vi "dcs_rtl_visv2.vi"() -> ()   [LabVIEW 2020]
uses:
  <vilib>/Utility/file.llb/Read Delimited Spreadsheet (DBL).vi
panel:
  out "Waveform Chart":cluster{dbl, dbl}(graph)
  out "1-D Array of Real":dbl[](array[numeric])
  out "size(s) 2":i32
  in  "milliseconds to wait":u32
  out "size(s) 4":i32[](array[numeric])
  out "Numeric":i32
  out "concatenated string":string
  out "size(s)":i32
  out "filenames":string[](array[string])
  in  "file path (dialog if empty) 2":path
  out "all rows 2":dbl[][](array[numeric])
  out "Waveform Graph 2":dbl[][](graph)
  out "Waveform Graph":dbl[][](graph)
  out "all rows":dbl[][](array[numeric])
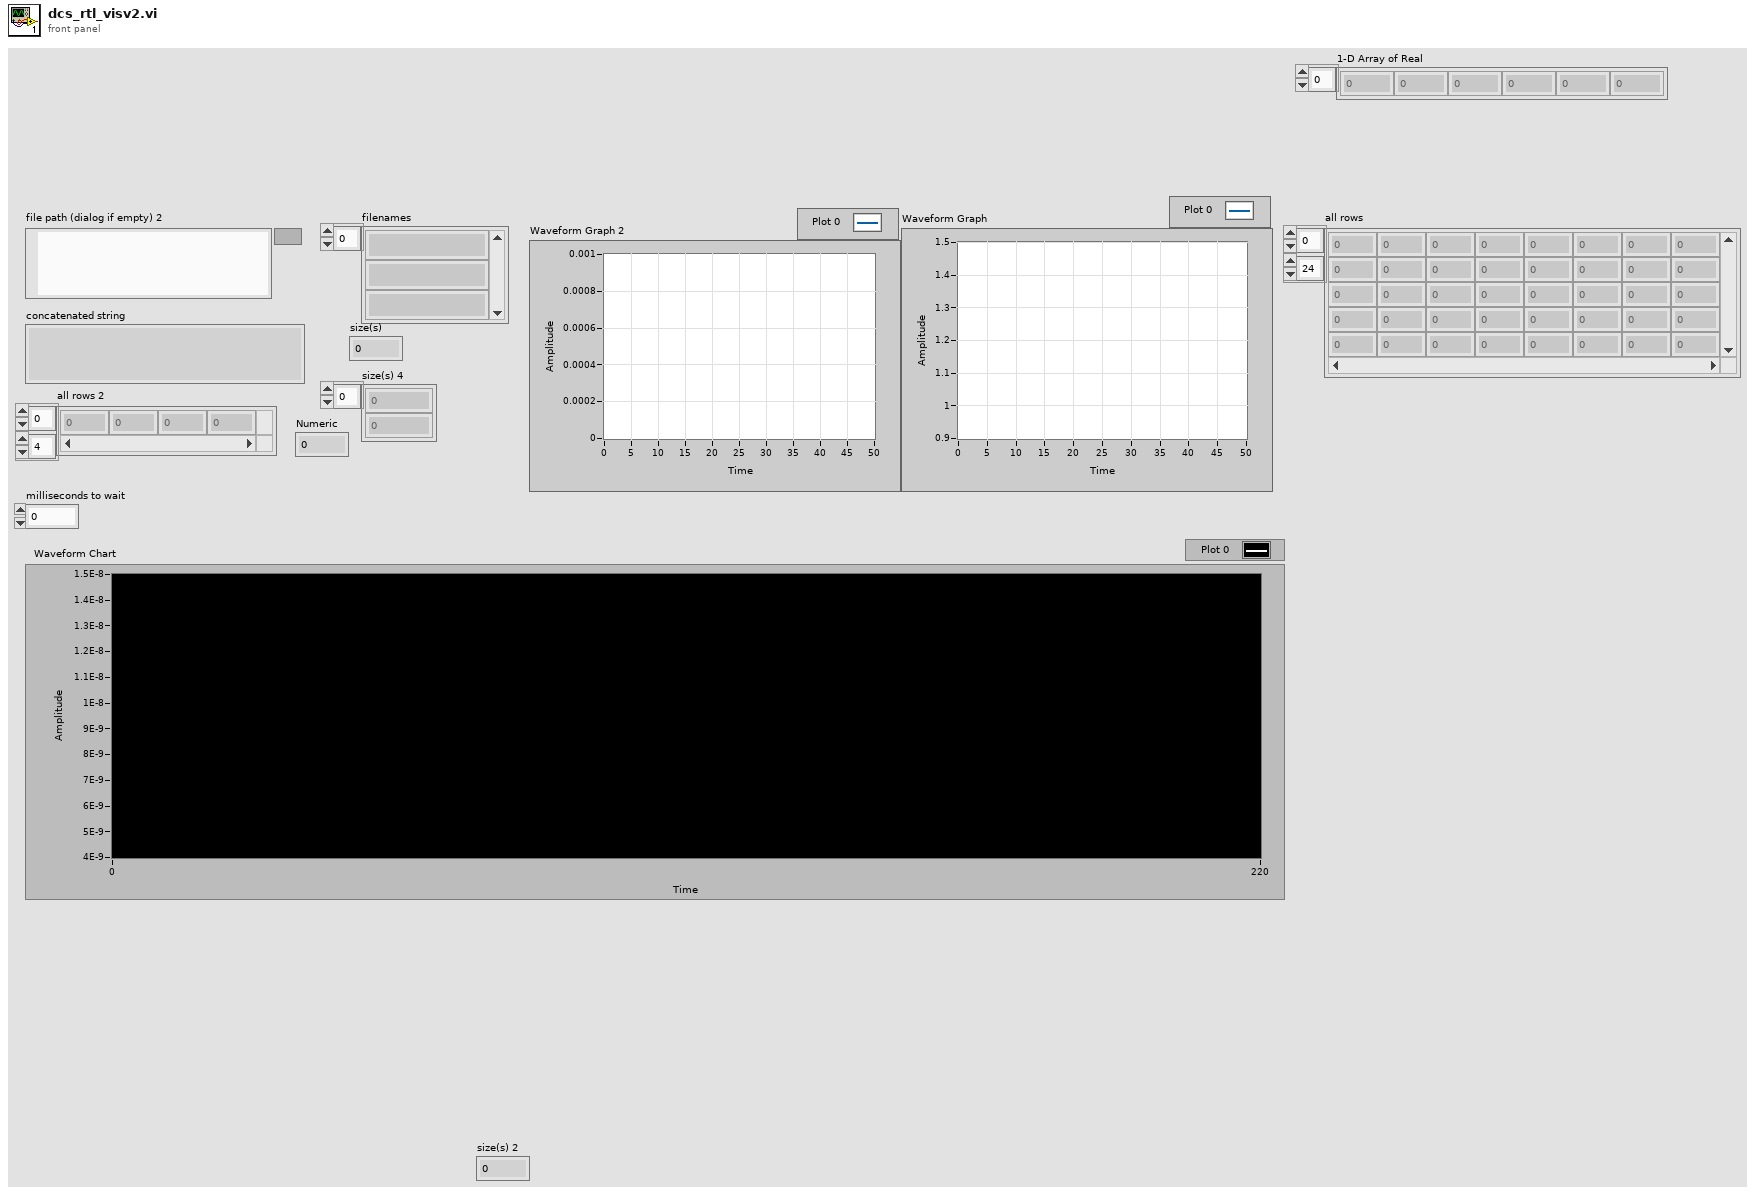
[diagram p1: front panel]
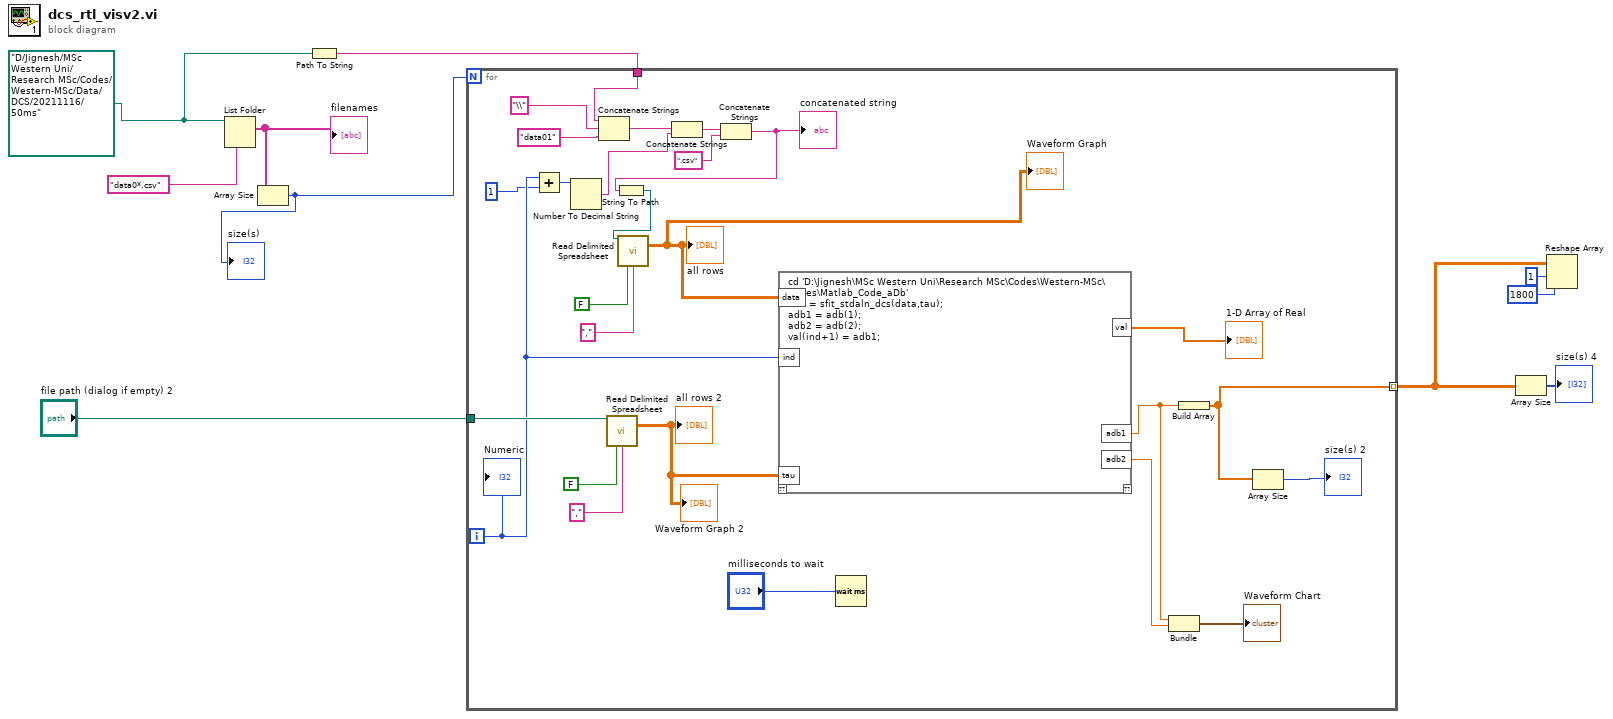
[diagram p0: block diagram]
diagram:
  w7 = path "D:/Jignesh/MSc Western Uni/Research MSc/Codes/Western-MSc/Data/DCS/20211116/50ms"
  n1 = List Folder(path=w7, pattern="data0*.csv") -> (filenames=w9:string[])  [unwired: 2 in, 3 out]
  "filenames" <- w9
  n2 = Array Size(array=w9) -> (size(s)=w6:i32)
  "size(s)" <- w6
  n3 = Path To String(path=w7) -> (string=w8:string)
  n4 = for {
    N: w6 -> [_]
    tunnel: "file path (dialog if empty) 2" -> [w32]
    tunnel: w8 -> [w28]
    tunnel: [w26] -> w4 mode=indexing
    i -> [w16]
    n5 = Add(x=w16, y=1) -> (x+y=w14:i32)
    n6 = Number To Decimal String(number=w14) -> (decimal integer string=w17:string)  [unwired: 1 in]
    n7 = Concatenate Strings(w28, "\\" ("string"), "data01" ("string")) -> (w27:string)
    n8 = call-poly <vilib>:"Read Delimited Spreadsheet.vi"("file path (dialog if empty)"=w32, "transpose? (F)"=FALSE, "delimiter (\\t)"="," ("delimiter (\\t)")) -> ("all rows"=w31:dbl[][])  [unwired: 7 in, 5 out]
    "all rows 2" <- w31
    "Waveform Graph 2" <- w31
    n9 = Concatenate Strings(w27, w17) -> (w13:string)
    n10 = Concatenate Strings(w13, ".csv" ("string")) -> (w12:string)
    "concatenated string" <- w12
    n11 = String To Path(string=w12) -> (path=w29:path)
    n12 = call-poly <vilib>:"Read Delimited Spreadsheet.vi"("file path (dialog if empty)"=w29, "transpose? (F)"=FALSE, "delimiter (\\t)"="," ("delimiter (\\t)")) -> ("all rows"=w30:dbl[][])  [unwired: 7 in, 5 out]
    "all rows" <- w30
    "Waveform Graph" <- w30
    n13 = script code="cd 'D:\\Jignesh\\MSc Western Uni\\Research MSc\\Codes\\Western-MSc\\Codes\\Matlab_Code_aDb'\nadb = sfit_stdaln_dcs(data,tau);\nadb1 = adb(1);\nadb2 = adb(2);\nval(ind+1) = adb1;"("data"=w30, "tau"=w31, "ind"=w16) -> ("adb1"=w21:dbl, "val"=→"1-D Array of Real":dbl[], "adb2"=w20:dbl)  [unwired: 1 in, 1 out]
    n14 = Wait (ms)(milliseconds to wait="milliseconds to wait") -> ()  [unwired: 1 out]
    n15 = Bundle(w21, w20) -> (→"Waveform Chart":cluster{dbl, dbl})  [unwired: 1 in]
    n16 = Build Array(w21) -> (w26:dbl[])
    n17 = Array Size(array=w26) -> (size(s)=→"size(s) 2":i32)
    "Numeric" <- w16
  }
  n18 = Array Size(array=w4) -> (size(s)=→"size(s) 4":i32[])
  n19 = Reshape Array(w4, 1 ("dimension size"), 1800 ("dimension size")) -> ()  [unwired: 1 out]
